vi "CreateWO-WordDocumentMain.vi"(7 "Work Order":string, 8 "error in":errorcluster, 11 "ERP-CreateWorkOrder in":refnum<class "ERP-CreateWorkOrder.lvclass">) -> (0 "error out":errorcluster, 2 "Word Doc Not Created":bool, 3 "ERP-CreateWorkOrder out":refnum<class "ERP-CreateWorkOrder.lvclass">)   [LabVIEW 2013, in "ERP-CreateWorkOrder.lvclass"]
uses:
  ERP-CreateWorkOrder.lvclass
  ERP-CreateWorkOrder.lvclass/ERP-CreateWorkOrder.ctl
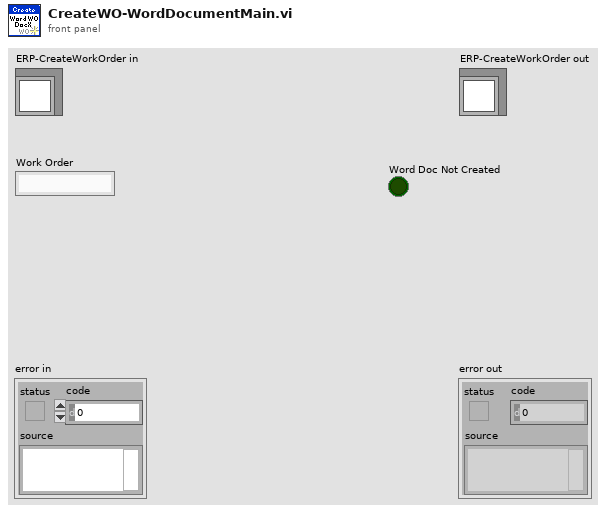
[diagram p1: front panel]
types:
  T1 = cluster{"Cert Yes or No":string, "Date Created":string, "Inspect":string, "Lot Number":string, "Manufacturer":string, "Customer":string, "Start Date":string, "Date Required":string, "Part Number":string, "Part Description":string, "Quantity":string, "Work Order":string, "Sales Order":string, "Shipper":string, "Special Instructions":string}
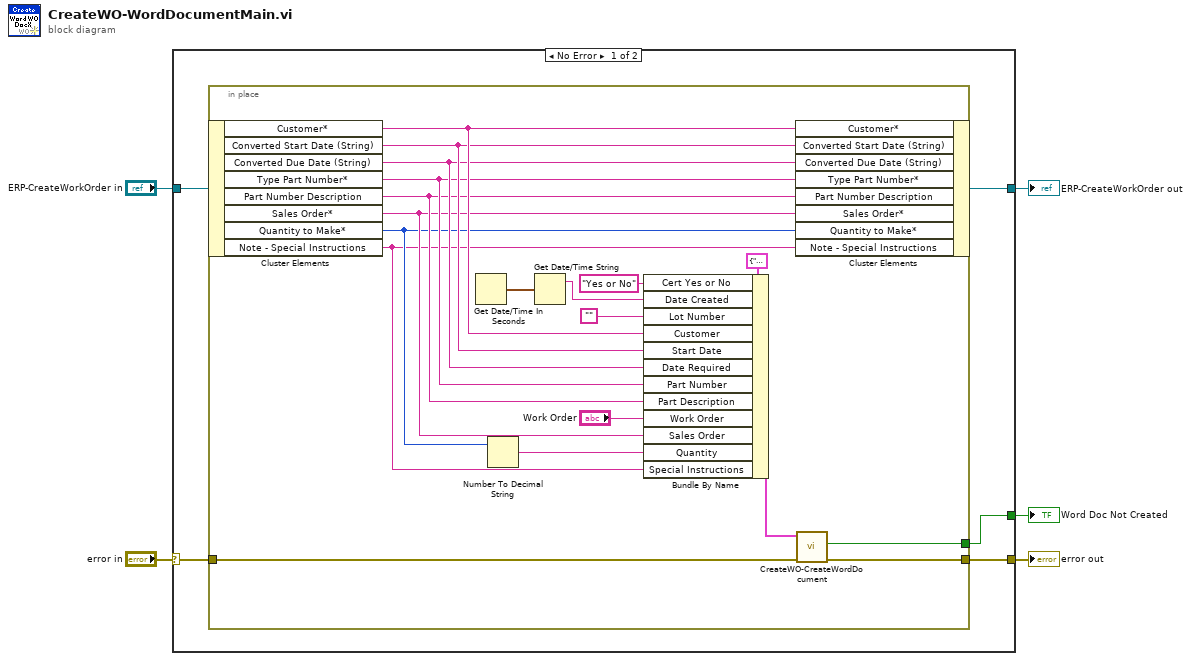
[diagram p0: block diagram]
diagram:
  n1 = case shown="No Error" "error in" {
    selector: "error in" -> [w10 w31]
    tunnel: [w9 w31] -> w4
    tunnel: [w6 w30] -> w2
    tunnel: "ERP-CreateWorkOrder in" -> [w7 w30]
    tunnel: [w8 _] -> w1
    frame No Error {
      n2 = in-place {
        in-place-border: w10 -> [w29]
        in-place-border: [w20] -> w9
        in-place-border: [w11] -> w8
        n3 = in-place-cluster #1(w7) -> ("Customer*"=w19:string, "Converted Start Date (String)"=w18:string, "Converted Due Date (String)"=w17:string, "Type Part Number*"=w16:string, "Part Number Description"=w15:string, "Sales Order*"=w14:string, "Quantity to Make*"=w13:i32, "Note - Special Instructions"=w12:string)
        n4 = Get Date/Time In Seconds() -> (seconds since 1Jan1904=w25:timestamp)
        n5 = Number To Decimal String(number=w13) -> (decimal integer string=w21:string)  [unwired: 1 in]
        n6 = Get Date/Time String(seconds (now)=w25) -> (date string=w24:string)  [unwired: 2 in, 1 out]
        n7 = Bundle By Name(cluster=T1 {"Cert Yes or No"="Testing Cert", "Date Created"="Date", "Inspect"="Inspect", "Lot Number"="Lot Number", "Manufacturer"="Manufactuer", "Customer"="Customer", "Start Date"="Due Date", "Date Required"="Date Required", "Part Number"="Part Number", "Part Description"="Part Descritption", "Quantity"="50", "Work Order"="Work Order", "Sales Order"="Work Order", "Shipper"="Shipper", "Special Instructions"="Special Instructions"} ("Input Word Cluster"), "Cert Yes or No"="Yes or No", "Date Created"=w24, "Lot Number"="", "Customer"=w19, "Start Date"=w18, "Date Required"=w17, "Part Number"=w16, "Part Description"=w15, "Work Order"="Work Order", "Sales Order"=w14, "Quantity"=w21, "Special Instructions"=w12) -> (w27:T1)
        n8 = in-place-cluster #1("Customer*"=w19, "Converted Start Date (String)"=w18, "Converted Due Date (String)"=w17, "Type Part Number*"=w16, "Part Number Description"=w15, "Sales Order*"=w14, "Quantity to Make*"=w13, "Note - Special Instructions"=w12) -> (w6:refnum<class "ERP-CreateWorkOrder.lvclass">)
        n9 = call "CreateWO-CreateWordDocument.vi"("error in"=w29, "Input Word Cluster"=w27) -> ("error out"=w20:errorcluster, "Word Doc Not Created"=w11:bool)  [unwired: 6 in, 1 out]
      }
    }
    frame Error {
    }
  }
  "error out" <- w4
  "ERP-CreateWorkOrder out" <- w2
  "Word Doc Not Created" <- w1
